vi "Class Casting.vi"(3 "Parent Label":string, 4 "Control Class":string, 5 "Parent Class":string) -> (0 "Add-on Label":string, 2 "Class":string)   [LabVIEW 2009]
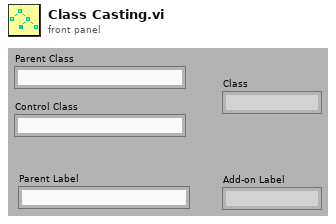
[diagram p1: front panel]
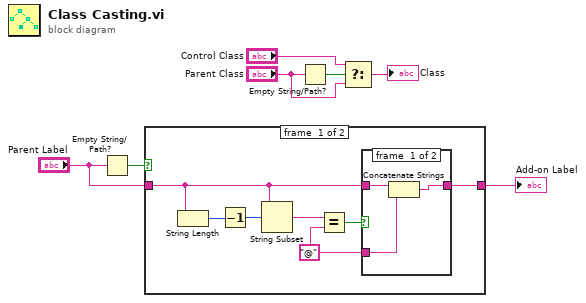
[diagram p0: block diagram]
diagram:
  n1 = Empty String/Path?(string/path="Parent Label") -> (empty?=w6:bool)
  n2 = case shown="False" w6 {
    tunnel: "Parent Label" -> [w13 w19]
    tunnel: [w14 w19] -> w1
    frame #0 {
      w8 = "@" ("string")
      n3 = String Length(string=w13) -> (length=w12:i32)
      n4 = Decrement(x=w12) -> (x-1=w11:i32)
      n5 = String Subset(string=w13, offset (0)=w11) -> (substring=w10:string)  [unwired: 1 out]
      n6 = Equal?(x=w10, y=w8) -> (x = y?=w9:bool)
      n7 = case shown="False" w9 {
        tunnel: [w17 w18] -> w14
        tunnel: w13 -> [w16 w18]
        tunnel: w8 -> [w15 _]
        frame #0 {
          n8 = Concatenate Strings(w16, w15) -> (w17:string)
        }
        frame #1 {
        }
      }
    }
    frame #1 {
    }
  }
  "Add-on Label" <- w1
  n9 = Empty String/Path?(string/path="Parent Class") -> (empty?=w7:bool)
  n10 = Select(t="Control Class", s=w7, f="Parent Class") -> (s? t:f=→"Class":string)
